vi "FactoryMethod.vi"(8 "error in (no error)":errorcluster, 11 "ConcreteCreatorA in":refnum<class "ConcreteCreatorA.lvclass">) -> (0 "error out":errorcluster, 2 "Product.":refnum<class "Product.lvclass">, 3 "ConcreteCreatorA out":refnum<class "ConcreteCreatorA.lvclass">)   [LabVIEW 2020, in "FactoryMethod.lvlib" / "ConcreteCreatorA.lvclass"]
uses:
  ConcreteCreatorA.lvclass
  Product/Product.lvclass
  ConcreteProductA/ConcreteProductA.lvclass
  E:/GitHub/Design-Patterns-GoF_-_NI-LV/Creational/FactoryMethod/Base_Example/ConcreteCreatorB/Product/Product.lvclass
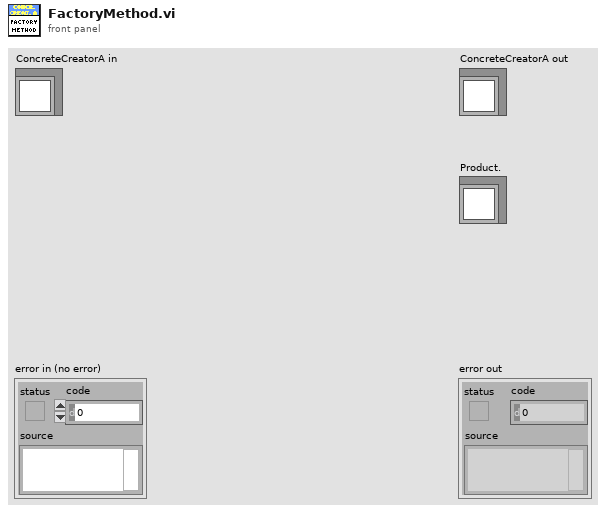
[diagram p1: front panel]
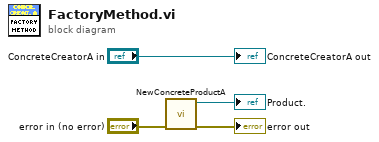
[diagram p0: block diagram]
diagram:
  n1 = call "NewConcreteProductA.vi"("error in (no error)"="error in (no error)") -> ("error out"=→"error out":errorcluster, "ConcreteProductA out"=→"Product.":refnum<class "ConcreteProductA.lvclass">)  [unwired: 9 in]
  "ConcreteCreatorA out" <- "ConcreteCreatorA in"
